vi "SetBase.vi"(7 "Actor":refnum<class "Actor.lvclass">, 11 "Base":T1) -> (5 "Actor":refnum<class "Actor.lvclass">)   [LabVIEW 2020, in "jettl.lvlib" / "Actor.lvclass"]
uses:
  Actor.lvclass
  Lifecycle.ctl
  jettl.lvlib
  Msg/Msg.lvclass
  MsgSet.ctl
  Msg.ctl
  Unified.ctl
  ChildUnifiedMap.ctl
  Base.ctl
  PostSetup.ctl
  PreSetup.ctl
  State.ctl
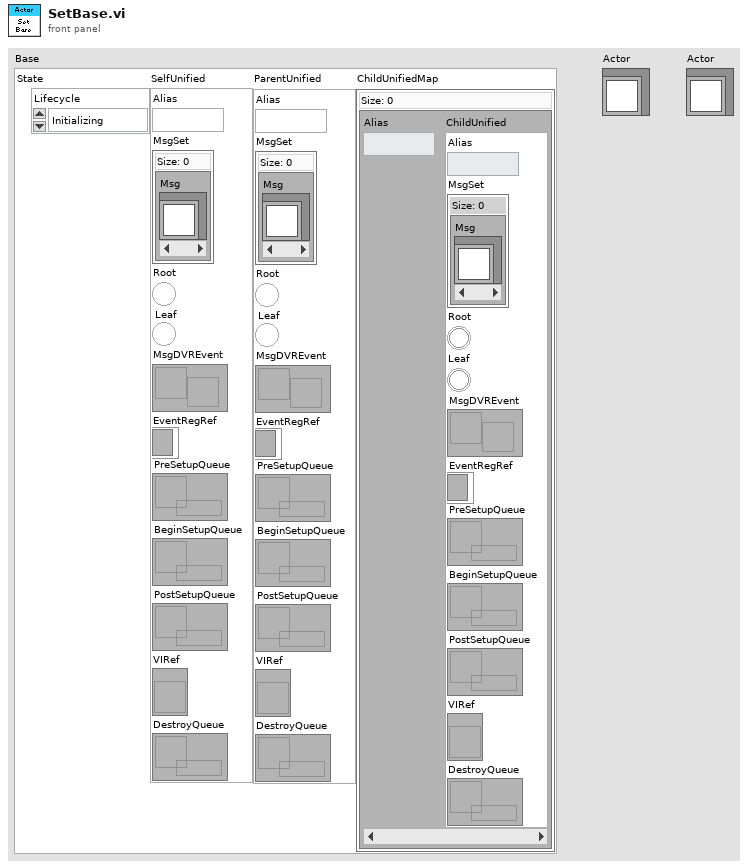
[diagram p1: front panel]
types:
  T1 = typedef "jettl.lvlib/Base.ctl" = cluster{"State":T2, "SelfUnified":T4, "ParentUnified":T4, "ChildUnifiedMap":T6}
  T2 = typedef "jettl.lvlib/State.ctl" = cluster{"Lifecycle":T3}
  T3 = typedef "jettl.lvlib/Lifecycle.ctl" = enum16{"Initializing", "SettingUp", "Starting", "Running", "Stopping", "TearingDown", "Terminated"}
  T4 = typedef "jettl.lvlib/Unified.ctl" = cluster{"Alias":string, "MsgSet":T5, "Root":bool, "Leaf":bool, "MsgDVREvent":refnum<user-event>, "EventRegRef":refnum<event-registration>, "PreSetupQueue":refnum<queue>, "BeginSetupQueue":refnum<queue>, "PostSetupQueue":refnum<queue>, "VIRef":refnum<vi>, "DestroyQueue":refnum<queue>}
  T5 = typedef "jettl.lvlib/MsgSet.ctl" = set{refnum<class "Msg.lvclass">}
  T6 = typedef "jettl.lvlib/ChildUnifiedMap.ctl" = map{string, T4}
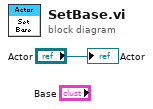
[diagram p0: block diagram]
diagram:
  "Actor" <- "Actor"
